vi "INI Extract Ring Text.vi"(0 "INI Extensions In":T1={"Type Descriptions Path"=path "Inifile Extensions/TypeDescriptions.ini", "Pre-Defined Type Names"=[], "Pre-Defined Type Info"=[], "Text Lists"=[]}, 11 "Error In (no error)":errorcluster) -> (4 "INI Extensions Out":T1={"Type Descriptions Path"=path "Inifile Extensions/TypeDescriptions.ini", "Pre-Defined Type Names"=[], "Pre-Defined Type Info"=[], "Text Lists"=[]}, 15 "Error Out":errorcluster)   [LabVIEW 2011]
doc: "This routine is used to initialize the globals with type information gathered from the controls registry. The controls registry should be used to pre-define all enumerated types such that they may be interpreted by the *.ini file management system. To register enumerated types for a component (Instrument driver, test, etc.), create a vi named ET REG 'Component'.vi, and place it in the controls registry directory. This vi should contain nothing more than the enumerated types. The names (labels) of these enumerated types will determine how they must be defined in the *.ini files. In the description column (3rd) of the *.ini file, only the name (label) of the enumerated type should appear, exactly as it appears in the controls registry."
uses:
  Type Defs/INI Extensions Cluster.ctl
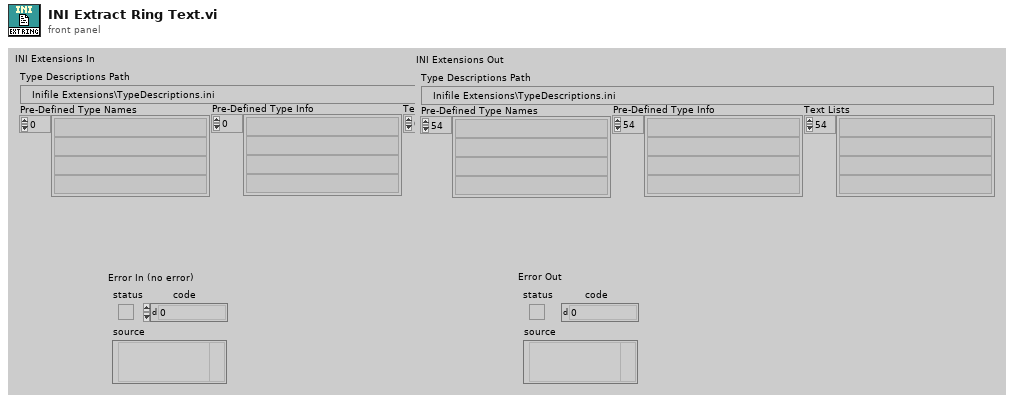
[diagram p1: front panel]
types:
  T1 = typedef "INI Extensions Cluster.ctl" = cluster{"Type Descriptions Path":path, "Pre-Defined Type Names":string[], "Pre-Defined Type Info":string[], "Text Lists":string[]}
  T2 = cluster{"name":string, "type desc":i16[], "flat data":string}[]
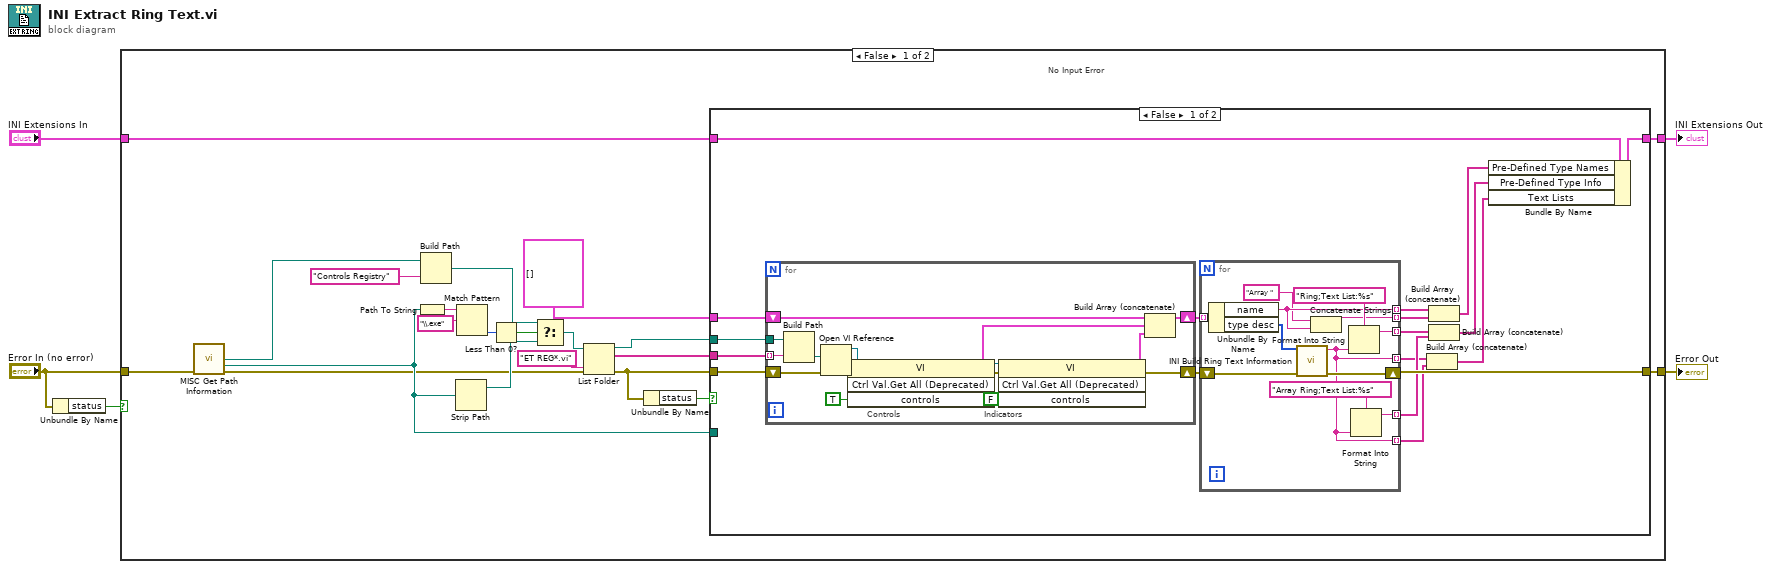
[diagram p0: block diagram]
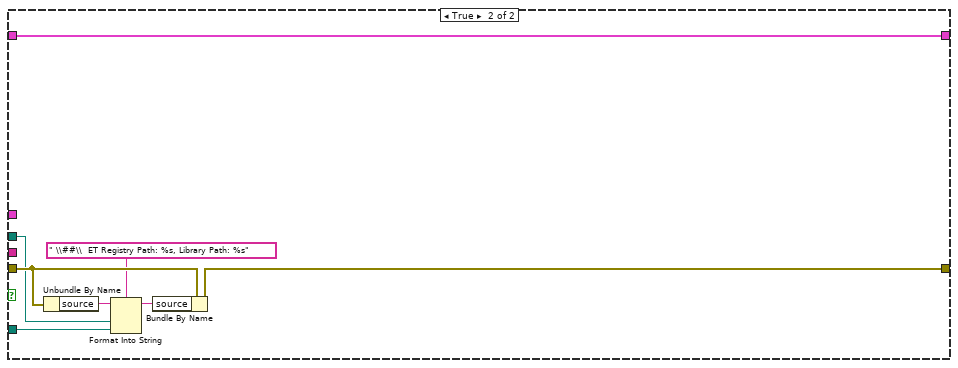
[diagram p2: hidden frame]
diagram:
  n1 = Unbundle By Name("Error In (no error)") -> ("status"=w5:bool)
  n2 = case shown="False" w5 {
    tunnel: [w23 w80] -> w4
    tunnel: "INI Extensions In" -> [w26 w81]
    tunnel: [w25 w81] -> w2
    tunnel: "Error In (no error)" -> [w9 w80]
    frame False {
      # "No Input Error"
      n3 = call "MISC Get Path Information.vi"("Error In (no error)"=w9) -> ("Support Directory"=w6:path, "Top Level VI Path"=w8:path, "Error Out"=w7:errorcluster)  [unwired: 12 out]
      n4 = Path To String(path=w8) -> (string=w13:string)
      n5 = Build Path(base path=w6, name or relative path="Controls Registry") -> (appended path=w19:path)
      n6 = Strip Path(path=w8) -> (stripped path=w14:path)  [unwired: 1 out]
      n7 = Match Pattern(string=w13, regular expression="\\.exe") -> (offset past match=w10:i32)  [unwired: 4 out]
      n8 = Less Than 0?(x=w10) -> (x < 0?=w11:bool)
      n9 = Select(t=w19, s=w11, f=w14) -> (s? t:f=w20:path)
      n10 = List Folder(path=w20, pattern="ET REG*.vi", error in=w7) -> (path out=w17:path, filenames=w18:string[], error out=w16:errorcluster)  [unwired: 2 out]
      n11 = Unbundle By Name(w16) -> ("status"=w15:bool)
      n12 = case shown="False" w15 {
        tunnel: w26 -> [w44 w79]
        tunnel: [w43 w79] -> w25
        tunnel: T2 [] -> [w42 _]
        tunnel: [w39 w77] -> w23
        tunnel: w16 -> [w29 w78]
        tunnel: w18 -> [w28 _]
        tunnel: w17 -> [w27 w73]
        tunnel: w8 -> [_ w72]
        frame False {
          n13 = for {
            shift-right: [w59] -> w40
            shift-left: w29 -> [w69]
            tunnel: w28 -> [w70] mode=indexing
            tunnel: w27 -> [w71]
            shift-right: [w62] -> w41
            shift-left: w42 -> [w63]
            # "Indicators"
            # "Controls"
            n14 = Build Path(base path=w71, name or relative path=w70) -> (appended path=w68:path)
            n15 = Open VI Reference(vi path=w68, error in (no error)=w69) -> (vi reference=w66:refnum<vi>, error out=w67:errorcluster)  [unwired: 4 out]
            n16 = invoke class="VI" method="Ctrl Val.Get All (Deprecated)"(reference=w66, error in=w67, "controls"=TRUE) -> (reference out=w61:refnum<vi>, error out=w60:errorcluster, "Get All Control Values"=w64:T2)  [unwired: 1 in, 1 out]
            n17 = invoke class="VI" method="Ctrl Val.Get All (Deprecated)"(reference=w61, error in=w60, "controls"=FALSE) -> (error out=w59:errorcluster, "Get All Control Values"=w58:T2)  [unwired: 1 in, 2 out]
            n18 = Build Array (concatenate)(w63, w64, w58) -> (w62:T2)
          }
          n19 = for {
            tunnel: w41 -> [w56] mode=indexing
            tunnel: [w47] -> w32 mode=indexing
            shift-right: [w54] -> w39
            shift-left: w40 -> [w55]
            tunnel: [w51] -> w37 mode=indexing
            tunnel: [w48] -> w36 mode=indexing
            tunnel: [w49] -> w38 mode=indexing
            tunnel: [w48] -> w35 mode=indexing
            tunnel: [w46] -> w30 mode=indexing
            n20 = Unbundle By Name(w56) -> ("name"=w47:string, "type desc"=w53:i16[])
            n21 = call "INI Build Ring Text Information.vi"("Type Descriptor"=w53, "Error In (no error)"=w55) -> ("Ring Text"=w48:string, "Error Out"=w54:errorcluster)  [unwired: 12 out]
            n22 = Concatenate Strings("Array " ("Substring"), w47) -> (w46:string)
            n23 = Format Into String(format string="Ring;Text List:%s" ("Format String"), w48) -> (resulting string=w51:string)  [unwired: 2 in, 1 out]
            n24 = Format Into String(format string="Array Ring;Text List:%s" ("Format String"), w48) -> (resulting string=w49:string)  [unwired: 2 in, 1 out]
          }
          n25 = Build Array (concatenate)(w36, w35) -> (w33:string[])
          n26 = Build Array (concatenate)(w32, w30) -> (w31:string[])
          n27 = Build Array (concatenate)(w37, w38) -> (w34:string[])
          n28 = Bundle By Name(cluster=w44, "Pre-Defined Type Names"=w31, "Pre-Defined Type Info"=w34, "Text Lists"=w33) -> (w43:T1)
        }
        frame True {
          n29 = Unbundle By Name(w78) -> ("source"=w75:string)
          n30 = Format Into String(format string=" \\##\\  ET Registry Path: %s, Library Path: %s", initial string=w75, w73, w72) -> (resulting string=w76:string)  [unwired: 1 in, 1 out]
          n31 = Bundle By Name(cluster=w78, "source"=w76) -> (w77:errorcluster)
        }
      }
    }
    frame True {
      # "Input Error"
    }
  }
  "Error Out" <- w4
  "INI Extensions Out" <- w2
